vi "chart legend set position.vi"(8 "error in (no error)":errorcluster, 10 "position":T1 items=["LXW_CHART_LEGEND_NONE", "LXW_CHART_LEGEND_RIGHT", "LXW_CHART_LEGEND_LEFT", "LXW_CHART_LEGEND_TOP", "LXW_CHART_LEGEND_BOTTOM", "LXW_CHART_LEGEND_TOP_RIGHT", "LXW_CHART_LEGEND_OVERLAY_RIGHT", "LXW_CHART_LEGEND_OVERLAY_LEFT"], 11 "chart":u32) -> (0 "error out":errorcluster)   [LabVIEW 2015, in "xlsxwriter.lvlib"]
doc: "void chart_legend_set_position(lxw_chart chart, uint8_t position);"
uses:
  xlsxwriter.lvlib
  Controls/lxw_chart_legend_position.ctl
  xlsxwriter.dll
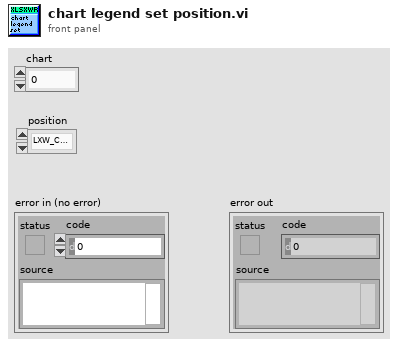
[diagram p1: front panel]
types:
  T1 = typedef "lxw_chart_legend_position.ctl" = u8
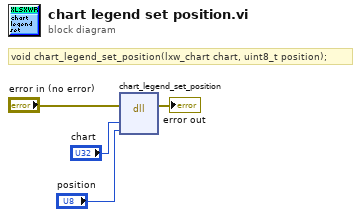
[diagram p0: block diagram]
diagram:
  # "void chart_legend_set_position(lxw_chart chart, uint8_t position);"
  n1 = dll-call lib="C:/Users/WDAGUtilityAccount/Desktop/Labview_Example-win32/xlsxwriter.*" fn="chart_legend_set_position"(error in="error in (no error)", "chart"="chart", "position"="position") -> (error out=→"error out":errorcluster)  [unwired: 5 in, 1 out]
